vi "SystemCheckState.vi"(8 "error in (no error)":errorcluster, 11 "Actual Start [i]":i64) -> (0 "error out":errorcluster, 2 "Cluster":T1, 3 "Numeric":i64)   [LabVIEW 2018]
uses:
  Type_Def/Type_Def Actuator Controls.ctl
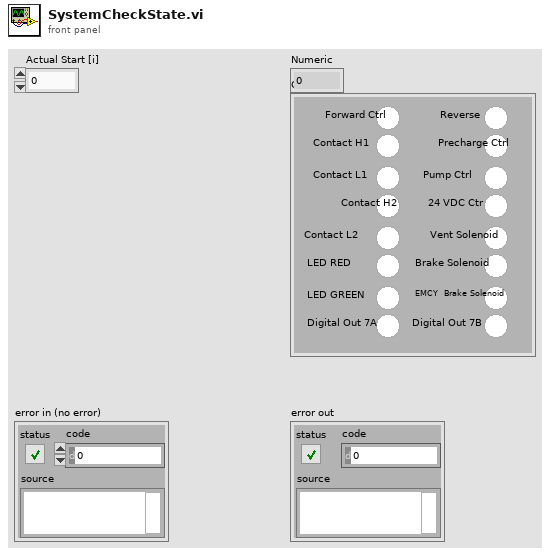
[diagram p1: front panel]
types:
  T1 = typedef "Type_Def Actuator Controls.ctl" = cluster{"Reverse ":bool, "Precharge Ctrl":bool, "Pump Ctrl":bool, "24 VDC Ctr":bool, "Vent Solenoid":bool, "Brake Solenoid":bool, "EMCY  Brake Solenoid":bool, "Digital Out 7B ":bool, "Forward Ctrl":bool, "Contact H1":bool, "Contact L1":bool, "Contact H2":bool, "Contact L2 ":bool, "LED RED":bool, "LED GREEN":bool, " Digital Out 7A":bool}
  T2 = cluster{"Forward":bool, "Low Side":bool, "Precharge":bool, "High Side":bool, "Digital Out 5":bool, "Digital Out 6":bool, "Digital Out 7 ":bool, "24 Power":bool, "Tank Valve ":bool, "Brake Valve":bool, "Pump":bool, "Digital Out 1 ":bool, "Digital Out 2":bool, "Digital Out 3":bool, "Digital Out 4 ":bool, "Reverse":bool}
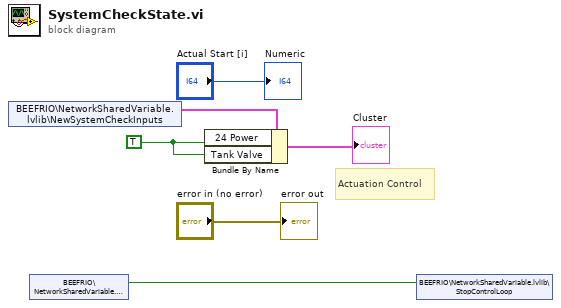
[diagram p0: block diagram]
diagram:
  w2 = TRUE
  # "Actuation Control"
  n1 = shared-variable "BEEFRIO\\NetworkSharedVariable.lvlib\\NewSystemCheckInputs"() -> (w4:T2)  [unwired: 1 in, 1 out]
  n2 = shared-variable "BEEFRIO\\NetworkSharedVariable.lvlib\\Shutdown"() -> (w1:bool)  [unwired: 1 in, 1 out]
  n3 = Bundle By Name(cluster=w4, "24 Power"=w2, "Tank Valve"=w2) -> (→"Cluster":T2)
  n4 = shared-variable "BEEFRIO\\NetworkSharedVariable.lvlib\\StopControlLoop"(w1) -> ()  [unwired: 1 in, 1 out]
  "error out" <- "error in (no error)"
  "Numeric" <- "Actual Start [i]"
